vi "read_ini_file_SCM_Pri_Limit.vi"(8 "error in (no error)":errorcluster, 9 "key":string="UUTFWFilePath_Pri", 10 "section":string="MAS80W", 11 "configuration file path":path=path "C:/Project/SolaHD_FCT/Configuration/config.ini") -> (0 "error out":errorcluster, 1 "found?":bool=TRUE, 2 "string":string)   [LabVIEW 2016]
uses:
  <vilib>/Utility/config.llb/Read Key (Path).vi
  <vilib>/Utility/config.llb/NI_LVConfig.lvlib
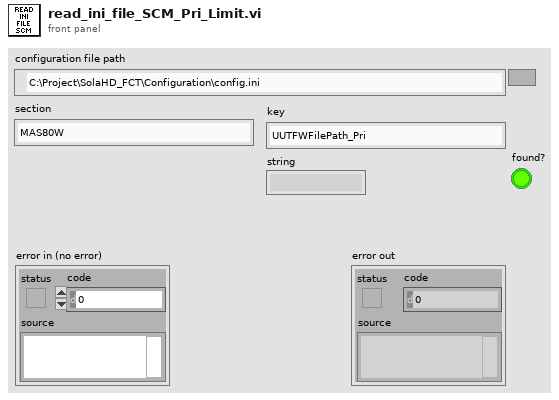
[diagram p1: front panel]
types:
  T1 = typedef "NI_LVConfig.lvlib/Config Data RefNum.ctl" = refnum<k1>
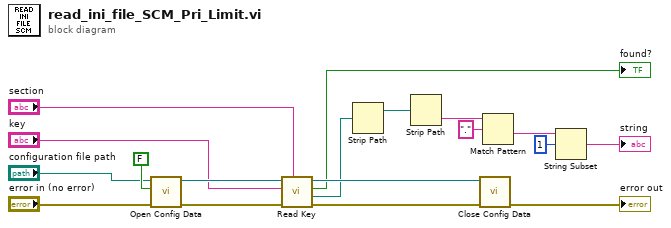
[diagram p0: block diagram]
diagram:
  n1 = call <vilib>:"Open Config Data.vi"("error in (no error)"="error in (no error)", "create file if necessary (T)"=FALSE, "configuration file path"="configuration file path") -> ("error out"=w13:errorcluster, "refnum"=w11:T1)  [unwired: 6 in, 1 out]
  n2 = call-poly <vilib>:"Read Key.vi"("section"="section", "error in (no error)"=w13, "key"="key", "refnum"=w11) -> ("error out"=w12:errorcluster, "value"=w7:path, "found?"=→"found?":bool, "refnum out"=w14:T1)  [unwired: 4 in]
  n3 = Strip Path(path=w7) -> (stripped path=w6:path)  [unwired: 1 out]
  n4 = Strip Path(path=w6) -> (name=w5:string)  [unwired: 1 out]
  n5 = call <vilib>:"Close Config Data.vi"("error in (no error)"=w12, "refnum"=w14) -> ("error out"=→"error out":errorcluster)  [unwired: 8 in, 1 out]
  n6 = Match Pattern(string=w5, regular expression=".") -> (after substring=w3:string)  [unwired: 1 in, 3 out]
  n7 = String Subset(string=w3, offset (0)=1) -> (substring=→"string":string)  [unwired: 1 in]
